vi "sound_to_fft.vi"(1 "Pure Sound":dynamicdata(graph)) -> (0 "FFT Out":dynamicdata(graph))   [LabVIEW 2024]
uses:
  <vilib>/express/express analysis/Spectral/Block/exnSpectralBlock spectral measurements peak poly.vi
  <vilib>/express/express analysis/Spectral/Block/exnSpectralBlock spectral measurements peak DDT.vi
  <vilib>/express/express analysis/Spectral/XNode/ExpressSpectralMeasurementsBlockNode.xnode
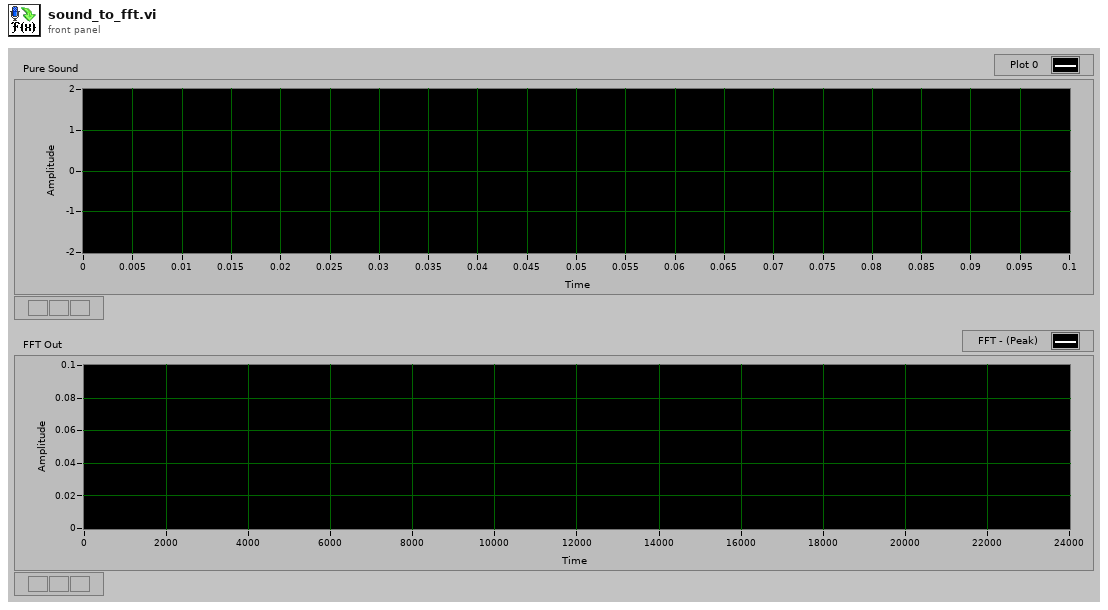
[diagram p1: front panel]
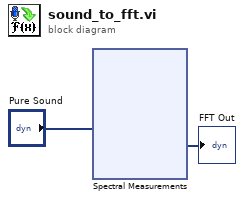
[diagram p0: block diagram]
diagram:
  n1 = xnode "Spectral Measurements"("Signals"="Pure Sound") -> ("FFT - (Peak)"=→"FFT Out":dynamicdata)  [unwired: 1 in, 2 out]
